vi "Create-Traj-Util-Test-Read-ini-file.vi"() -> ()   [LabVIEW 2019]
panel:
  in  "Tab Control":enum32{"Page 2", "Page 3", "Page 4", "Page 5"}(tab)
  out "read ini error":errorcluster
  in  "Field Selector":string(combo)
  out "FIeld Description":string
  out "error out 2":errorcluster
  out "read img err":errorcluster
  out "Disp Y Res":i32
  out "Disp X res":i32
  out "Org FIeld X res":dbl
  out "Org FIeld Y res":dbl
  out "Siized FIeld Y Res":i32
  out "Sized Field X res":i32
  out "new picture":picture
  out "Field Image":T1(plugin-control)
  out "new picture 2":picture
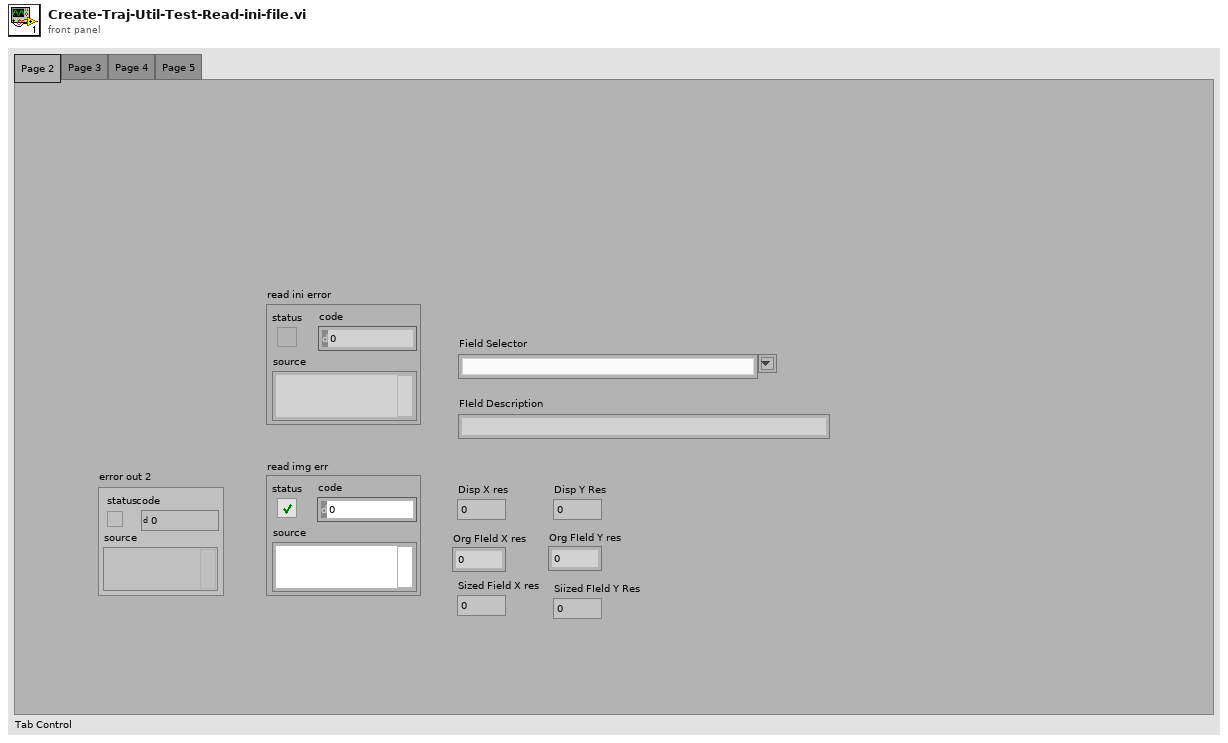
[diagram p1: front panel]
types:
  T1 = typedef "IMAQ Image.ctl" = refnum<image>
  T2 = typedef "Image Type" = u32
  T3 = typedef "TrajectoryUtils_Field_Info.ctl" = cluster{"FIeld_File_Name":string, "Top_Left_X":i32, "Top_Left_Y":i32, "Bottom_Right_X":i32, "Bottom_Right_Y":i32, "Field_Size_X":dbl, "Field_Size_Y":dbl, "FIeld_Size_Units":string}
  T4 = typedef "imagedata.ctl" = cluster{"image type":i32, "image depth":i32, "image":u8[], "mask":u8[], "colors":u32[], "Rectangle":cluster{"left":i16, "top":i16, "right":i16, "bottom":i16}}
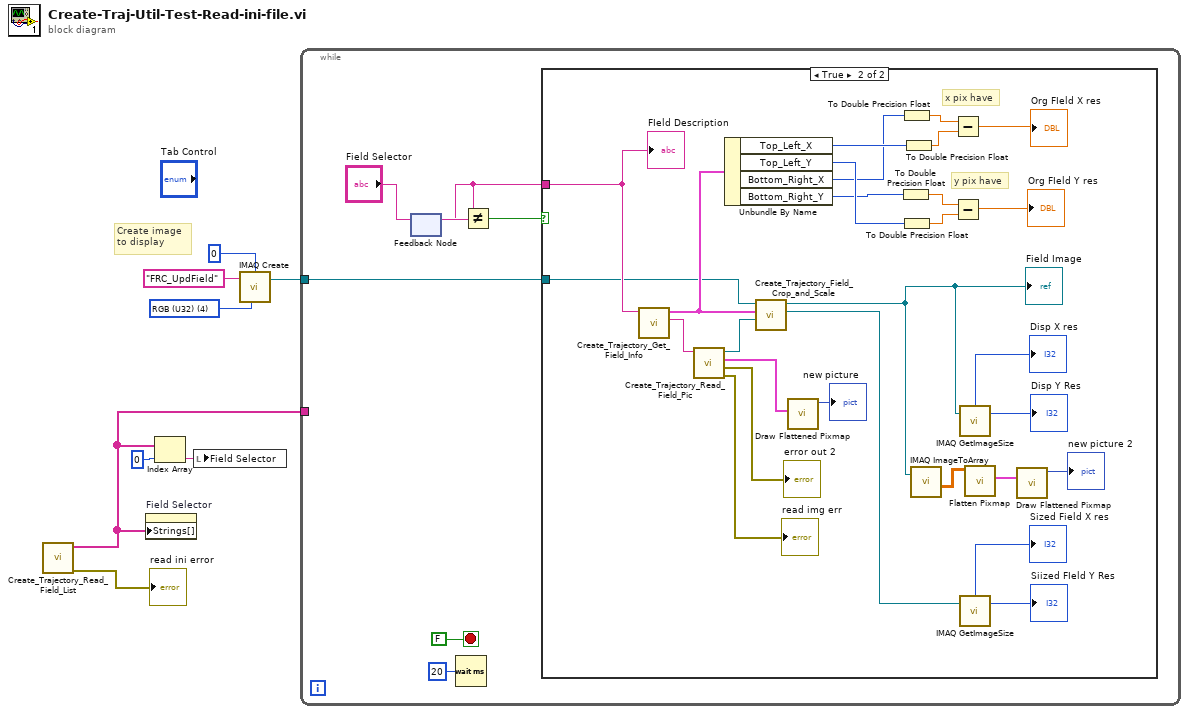
[diagram p0: block diagram]
diagram:
  w3 = T2 4 items=["Grayscale (U8)", "Grayscale (I16)", "Grayscale (SGL)", "Complex (CSG)", "RGB (U32)", "HSL (U32)", "RGB (U64)", "Grayscale (U16)"] ("Image Type")
  # "Create image \nto display"
  n1 = call "Create_Trajectory_Read_Field_List.vi"() -> ("error out"=→"read ini error":errorcluster, "section names"=w1:string[])  [unwired: 10 in]
  n2 = property on="Field Selector" class="CmbBox"("Strings[]"=w1) -> ()  [unwired: 2 in, 2 out]
  n3 = Index Array(array=w1, index=0) -> (element=w7:string)
  n4 = local write "Field Selector"(w7) -> ()
  n5 = call "IMAQ Create"("Border Size"=0, "Image Name"="FRC_UpdField", "Image Type"=w3) -> ("New Image"=w2:T1)  [unwired: 2 in, 1 out]
  n6 = while {
    tunnel: w2 -> [w9]
    tunnel: w1 -> [_]
    stop <- FALSE stop-if-true
    n7 = feedback-in #1("Field Selector") -> ()
    n8 = feedback #1() -> (w12:string)  [unwired: 1 in]
    n9 = Wait (ms)(milliseconds to wait=u32 20) -> ()  [unwired: 1 out]
    n10 = Not Equal?(x="Field Selector", y=w12) -> (x != y?=w10:bool)
    n11 = case shown="True" w10 {
      tunnel: "Field Selector" -> [_ w36]
      tunnel: w9 -> [_ w15]
      frame False {
      }
      frame True {
        # "y pix have"
        # "x pix have"
        n12 = call "Create_Trajectory_Get_Field_Info.vi"("Field Selector"=w36) -> ("value"=w16:string, "input cluster"=w21:T3)  [unwired: 9 in]
        n13 = call "Create_Trajectory_Read_Field_Pic.vi"("value"=w16) -> ("error out"=→"read img err":errorcluster, "error out 2"=→"error out 2":errorcluster, "image data"=w40:T4, "Refnum out"=w35:T1)  [unwired: 7 in]
        n14 = Unbundle By Name(w21) -> ("Top_Left_X"=w20:i32, "Top_Left_Y"=w19:i32, "Bottom_Right_X"=w18:i32, "Bottom_Right_Y"=w17:i32)
        n15 = call "Create_Trajectory_Field_Crop_and_Scale.vi"("Field Image"=w35, "field Info"=w21, "Display Image"=w15) -> ("FIeld Image Out"=w26:T1, "Disp Image Out"=w25:T1)  [unwired: 7 in]
        "Field Image" <- w25
        n16 = call <vilib>:"Draw Flattened Pixmap.vi"("image data"=w40) -> ("new picture"=→"new picture":picture)  [unwired: 8 in]
        n17 = To Double Precision Float(number=w17) -> (double precision float=w32:dbl)
        n18 = To Double Precision Float(number=w18) -> (double precision float=w33:dbl)
        n19 = To Double Precision Float(number=w19) -> (double precision float=w31:dbl)
        n20 = To Double Precision Float(number=w20) -> (double precision float=w34:dbl)
        n21 = call "IMAQ ImageToArray"("Image"=w25) -> ("Image Pixels (Float)"=w24:sgl[][])  [unwired: 2 in, 5 out]
        n22 = Subtract(x=w33, y=w34) -> (x-y=→"Org FIeld X res":dbl)
        n23 = Subtract(x=w32, y=w31) -> (x-y=→"Org FIeld Y res":dbl)
        n24 = call "IMAQ GetImageSize"("Image"=w25) -> ("Y Resolution"=→"Disp Y Res":i32, "X Resolution"=→"Disp X res":i32)  [unwired: 3 in, 1 out]
        n25 = call "IMAQ GetImageSize"("Image"=w26) -> ("Y Resolution"=→"Siized FIeld Y Res":i32, "X Resolution"=→"Sized Field X res":i32)  [unwired: 3 in, 1 out]
        n26 = call <vilib>:"Flatten Pixmap.vi"("24-bit pixmap"=w24) -> ("image data"=w23:T4)  [unwired: 5 in, 5 out]
        n27 = call <vilib>:"Draw Flattened Pixmap.vi"("image data"=w23) -> ("new picture"=→"new picture 2":picture)  [unwired: 1 in, 7 out]
        "FIeld Description" <- w36
      }
    }
  }
